vi "get_result.vi"(8 "error in":errorcluster, 10 "timeout ms":i32=10000, 11 "connection ID":refnum<k5>) -> (0 "error out":errorcluster, 1 "result":variant, 2 "JSON Tree":variant, 3 "connection ID out":refnum<k5>)   [LabVIEW 2010]
uses:
  globals.vi
  i3-json-1.0.0-10/JSON Parsing/Get Object Parameter Files/Get Object Parameter - Object.vi
  i3-json-1.0.0-10/i3-json.lvlib
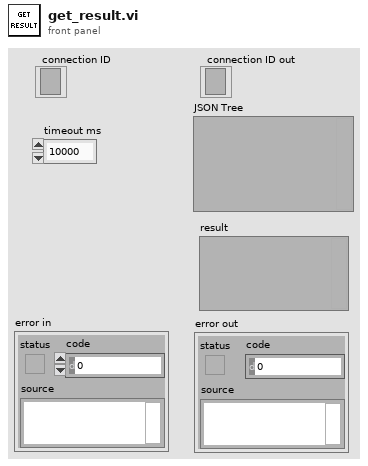
[diagram p1: front panel]
types:
  T1 = enum16{"Standard", "Buffered", "CRLF", "Immediate"}
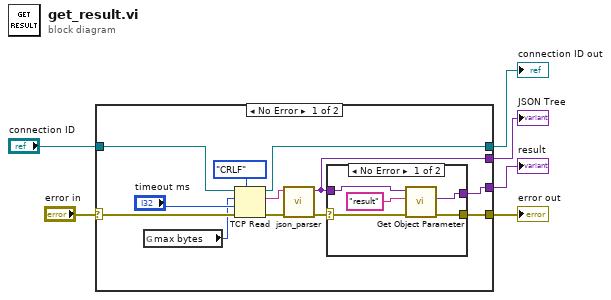
[diagram p0: block diagram]
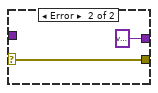
[diagram p2: hidden frame]
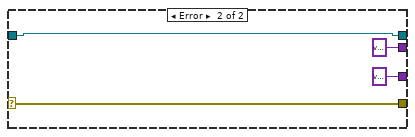
[diagram p3: hidden frame]
diagram:
  n1 = case shown="No Error" "error in" {
    selector: "error in" -> [w13 w29]
    tunnel: [w8 w29] -> w6
    tunnel: [w10 variant ("JSON Tree Out Passthrough")] -> w5
    tunnel: [w15 w27] -> w4
    tunnel: "connection ID" -> [w12 w27]
    tunnel: [w9 variant ("JSON Object")] -> w1
    frame No Error {
      n2 = global read "globals.vi" "max bytes"() -> (w7:i32)
      n3 = TCP Read(connection ID=w12, bytes to read=w7, error in (no error)=w13, 7:T1."CRLF" ("mode (standard)"), 9:"timeout ms") -> (connection ID out=w15:refnum<k5>, data out=w16:string, error out=w14:errorcluster)
      n4 = call "json_parser.vi"("error in"=w14, "JSON String"=w16) -> ("error out"=w11:errorcluster, "JSON Tree Out Passthrough"=w10:variant)  [unwired: 8 in]
      n5 = case shown="No Error" w11 {
        selector: w11 -> [w22 w25]
        tunnel: w10 -> [w21 _]
        tunnel: [w20 variant ("JSON Object")] -> w9
        tunnel: [w19 w25] -> w8
        frame No Error {
          n6 = call-poly "Get Object Parameter.vi"("error in (no error)"=w22, "Parameter Name"="result", "JSON Tree In (JSON Object)"=w21) -> ("error out"=w19:errorcluster, "JSON Object"=w20:variant)  [unwired: 5 in, 2 out]
        }
        frame Error {
        }
      }
    }
    frame Error {
    }
  }
  "error out" <- w6
  "JSON Tree" <- w5
  "connection ID out" <- w4
  "result" <- w1
